vi "Measurement UI.vi"() -> ()   [LabVIEW 2023, in "Single Tone_Class D Amplifier_UI.lvlib"]
uses:
  Single Tone_Class D Amplifier_UI.lvlib
  shared/controls/units - snr.ctl
  shared/controls/units - ratio.ctl
  shared/controls/digital output level units.ctl
  shared/ui/controls/view.ctl
  UI State.ctl
  <vilib>/Utility/miscctls.llb/LVBoundsTypeDef.ctl
  <vilib>/Utility/miscctls.llb/LVPoint32TypeDef.ctl
  <vilib>/Utility/miscctls.llb/LVPointTypeDef.ctl
  shared/ui/UI Helpers.lvlib
  shared/audio popup ui/Audio Popup UI.lvlib
  shared/controls/audio controls.lvlib
panel:
  in  "view legend":T1
  out "time domain":waveform(dbl)[](graph)
  out "frequency domain":cluster{"x0":dbl, "dx":dbl, "magnitude":dbl[]}[](graph)
  out "meas table":string[][](table)
  in  "digital serial cfg file":string
  out "output power (W)":dbl[](array[numeric])
  out "SFDR (dBc)":dbl[](array[numeric])
  out "gain":dbl[](array[numeric])
  out "dynamic range (dB)":dbl[](array[numeric])
  out "THD":dbl[](array[numeric])
  out "THD+N":dbl[](array[numeric])
  out "SNR":dbl[](array[numeric])
  out "phase (deg)":dbl[](array[numeric])
  out "amplitude (dBFS)":dbl[](array[numeric])
  out "amplitude (Vrms)":dbl[](array[numeric])
  out "frequency (Hz)":dbl[](array[numeric])
  out "channel names":string[](array[string])
  in  "Configuration tab":enum32{"Protocol", "Measurement", "Units"}(tab)
  out "digital serial file name":string
  in  "configure digital serial":bool
  in  "master clock channel list":string caption="Master Clock Channel"
  in  "digital channel list":string caption="Digital Audio Channel"
  in  "output level":dbl=-1.0 caption="Output level" format="%#_3f"
  in  "output level units":T2
  in  "min settling cycles":u32 caption="Minimum settling cycles"
  in  "min settling time (s)":dbl=0.1 caption="Minimum settling time" format="%#_6ps"
  in  "min measurement cycles":u32 caption="Minimum measurement cycles"
  in  "min measurement time (s)":dbl=0.1 caption="Minimum measurement time" format="%#_6ps"
  in  "Acquisition channel":tag
  in  "acq sampling rate":dbl=51200.0 caption="Sample rate" format="%#.6pHz"
  in  "lowpass filter":T3(ring) caption="Lowpass filter"
  in  "highpass filter":enum32{"DC", "AC"}(ring) caption="Highpass filter"
  in  "band start":dbl=20.0 caption="Band start" format="%#_6pHz"
  in  "band stop":dbl=20000.0 caption="Band stop" format="%#_6pHz"
  in  "weighting filter":T4(ring)=enum."A-weighting" caption="Weighting filter"
  in  "load impedance":dbl=4.0 caption="Load impedance" format="%#_6p Ohms"
  in  "output range (pk-pk)":dbl=15.0 caption="Output range" format="%.3p Vpk-pk"
  in  "signal frequency":dbl=1000.0 caption="Frequency" format="%#_6pHz"
  in  "gain units":T5 caption="Gain"
  in  "THD units":T5 caption="THD"
  in  "THD+N units":T5 caption="THD+N"
  in  "SNR units":T6 caption="SNR"
  in  "channel 0 offset":u32=1
  out "fft - data":dbl[](array[numeric])
  out "fft - df":dbl
  out "fft - f0":dbl
  out "wfm - data":dbl[](array[numeric])
  out "wfm - dt":dbl
  out "wfm - t0":dbl
  in  "acq channel":string="PXI1Slot4/ai0"
  in  "signal phase":dbl caption="phase"
  # "hidden controls - used to sync with MeasLink"
  # "hidden indicators"
  # "Digital Serial Settings"
  # "Harware Resource"
  # "Filters"
  # "Output"
  # "Acquisition"
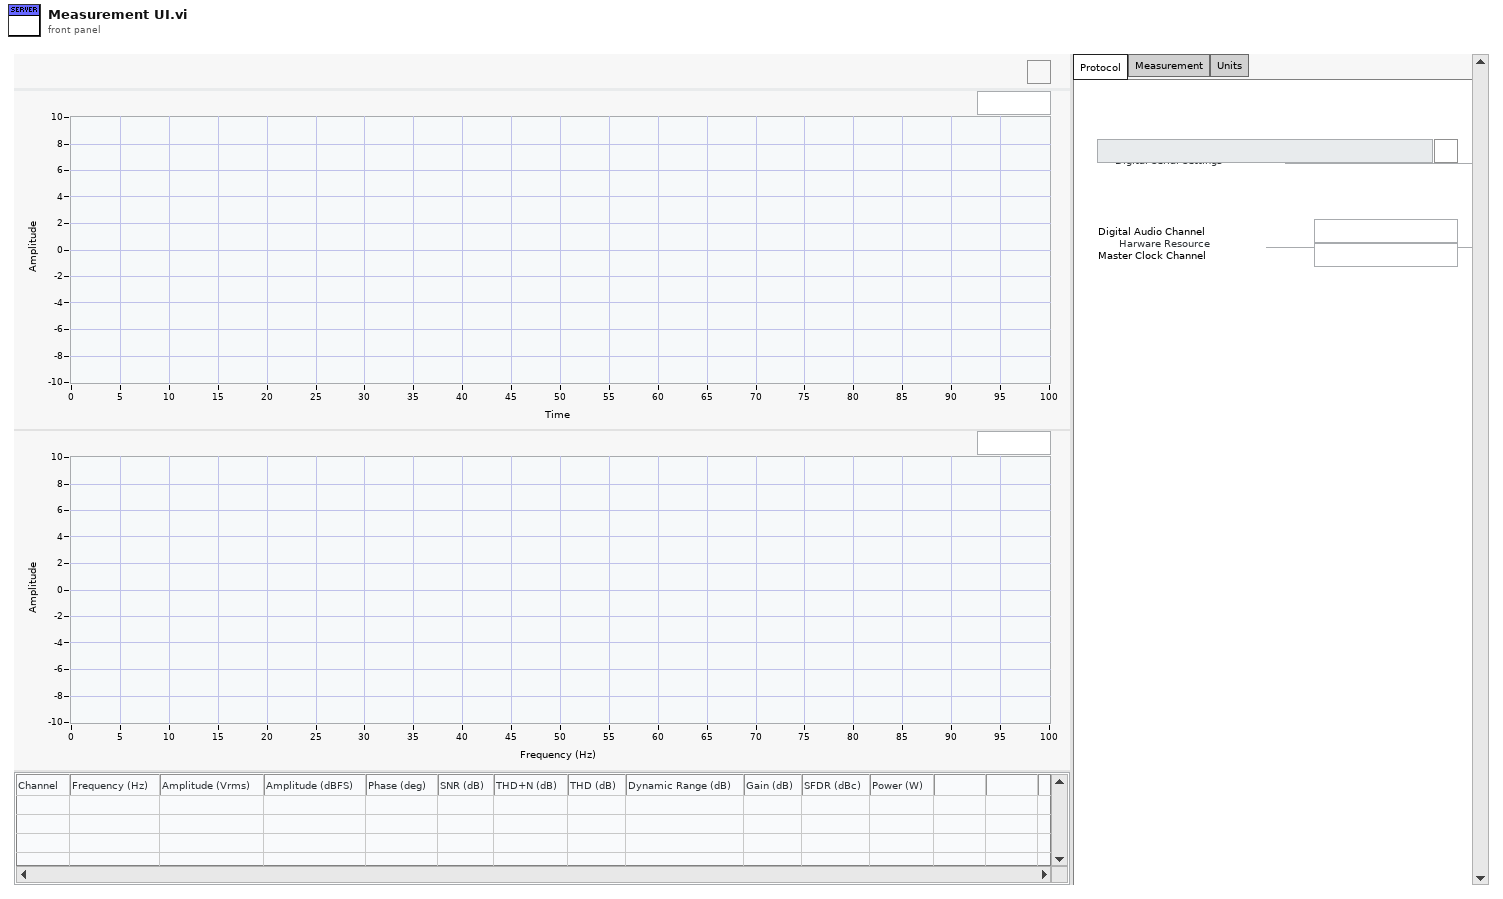
[diagram p1: front panel]
types:
  T1 = typedef "UI Helpers.lvlib/view.ctl" = bool
  T2 = typedef "audio controls.lvlib/digital output level units.ctl" = enum32{"% FS", "dBFS", "V"}
  T3 = enum32{"No filter", "AES17 20kHz", "AES17 40kHz"}
  T4 = enum32{"Linear", "A-weighting", "B-weighting", "C-weighting"}
  T5 = typedef "audio controls.lvlib/units - ratio.ctl" = enum32{"dB", "%", "x/y"}
  T6 = typedef "audio controls.lvlib/units - snr.ctl" = enum32{"dB", "x/y"}
  T7 = typedef "Single Tone_Class D Amplifier_UI.lvlib/UI State.ctl" = cluster{"Graph Size":T8, "Legend Visible":bool, "Mouse Coords":T9, "PostUI event occurred":bool, "digital serial cfg file":path}
  T8 = typedef "LVBoundsTypeDef.ctl" = cluster{"Width":u32, "Height":u32}
  T9 = typedef "LVPoint32TypeDef.ctl" = cluster{"Horizontal":i32, "Vertical":i32}
  T10 = typedef "LVPointTypeDef.ctl" = cluster{"Horizontal":i16, "Vertical":i16}
  T11 = typedef "Audio Popup UI.lvlib/audio settings.ctl" = cluster{"digital serial file":string}
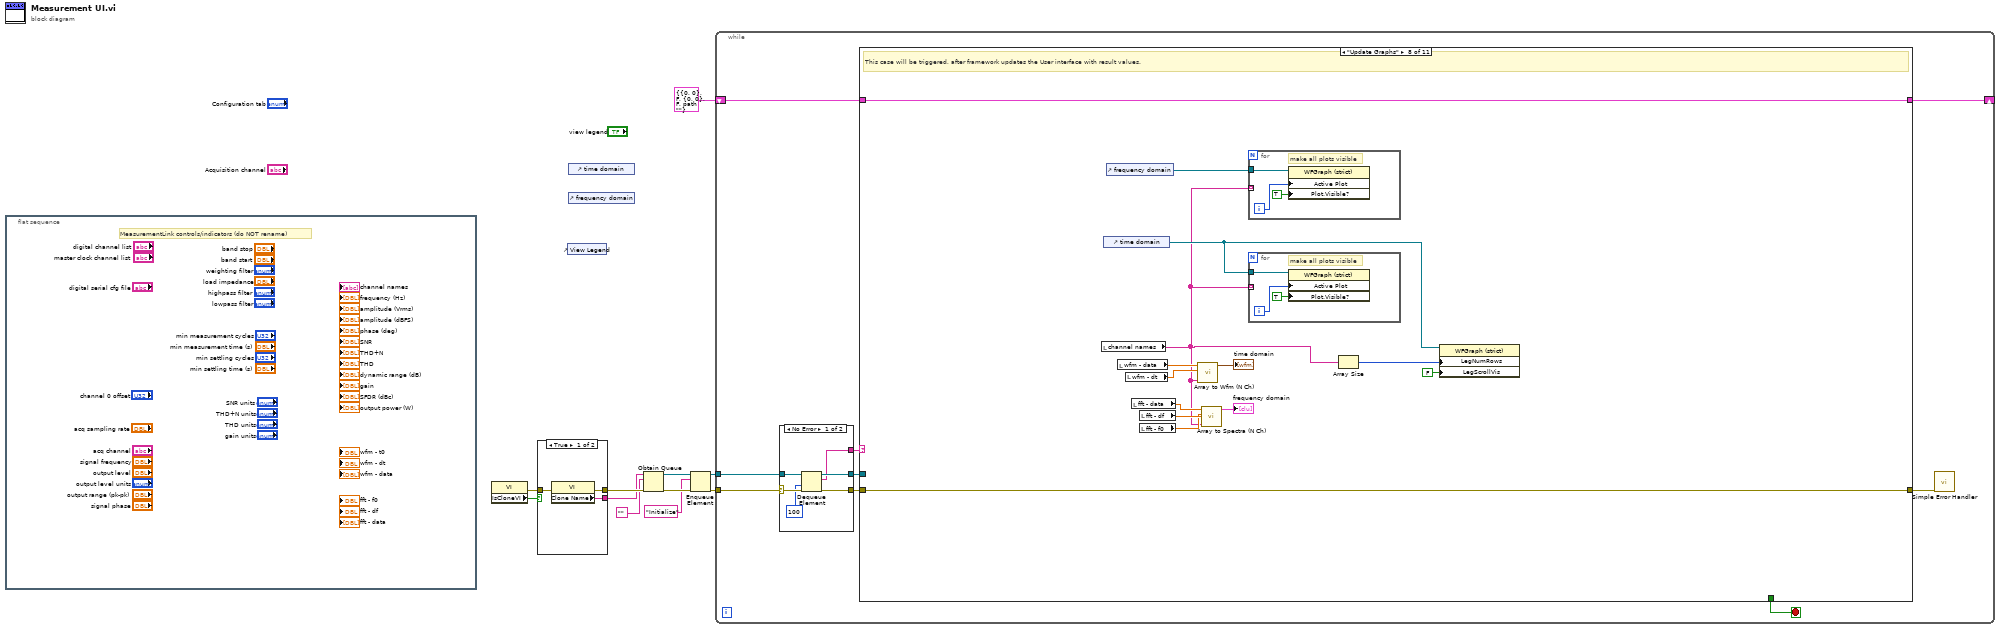
[diagram p0: block diagram]
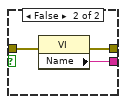
[diagram p2: hidden frame]
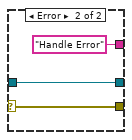
[diagram p3: hidden frame]
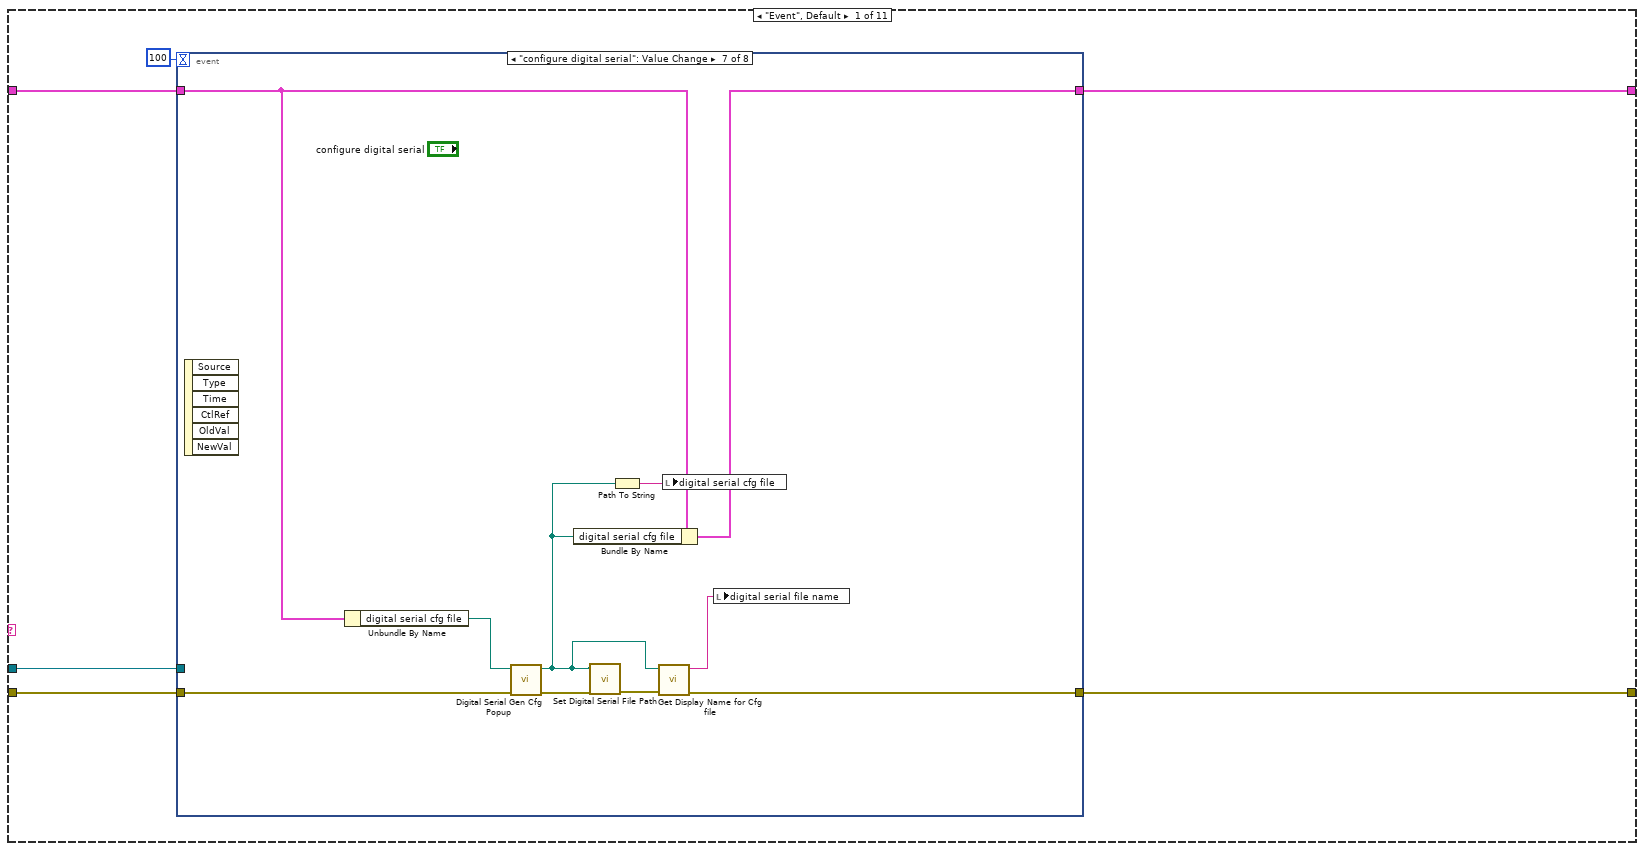
[diagram p4: hidden frame]
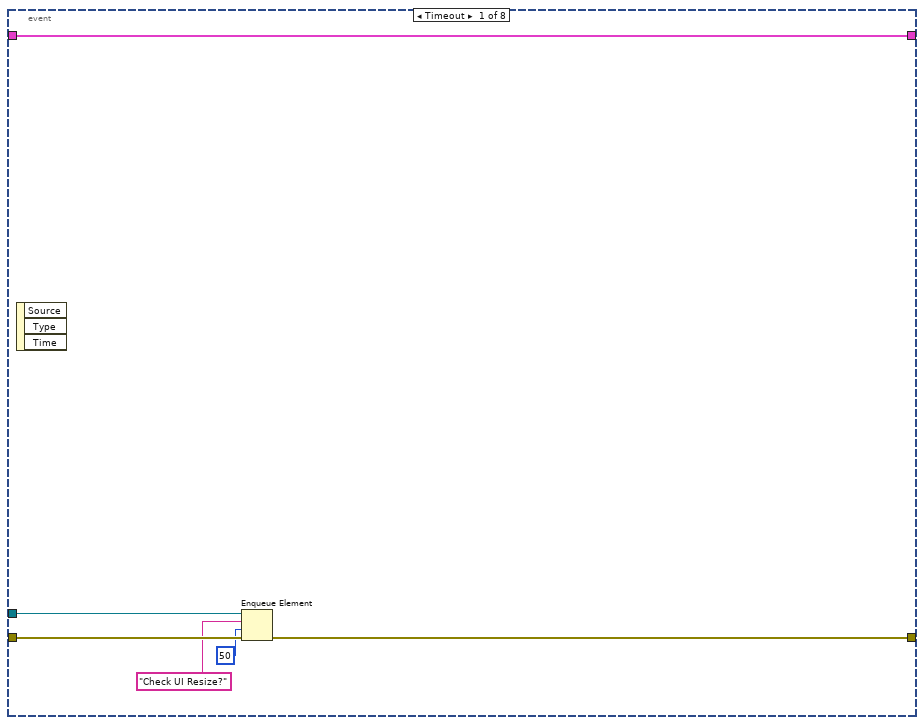
[diagram p5: hidden frame]
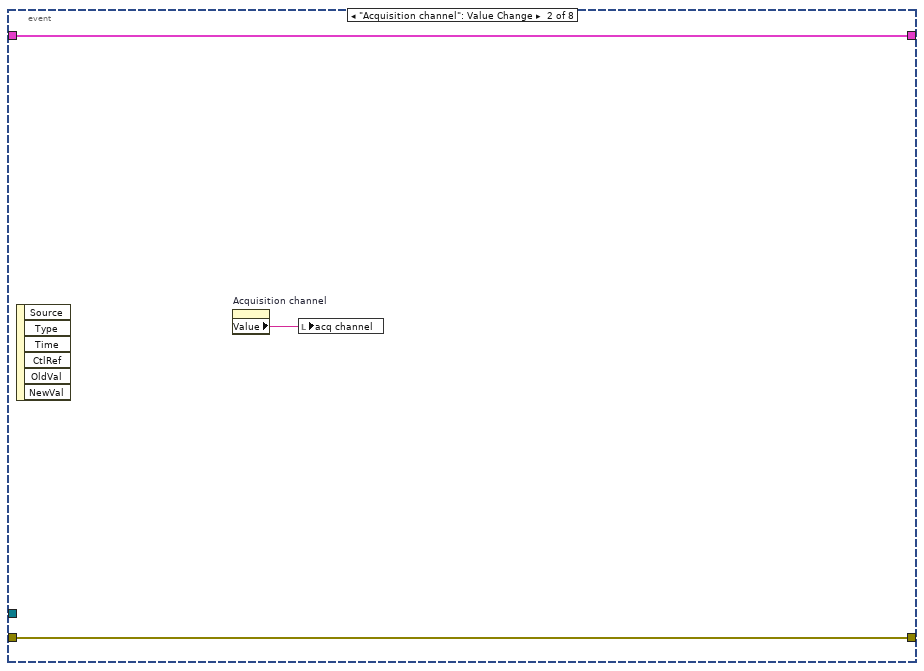
[diagram p6: hidden frame]
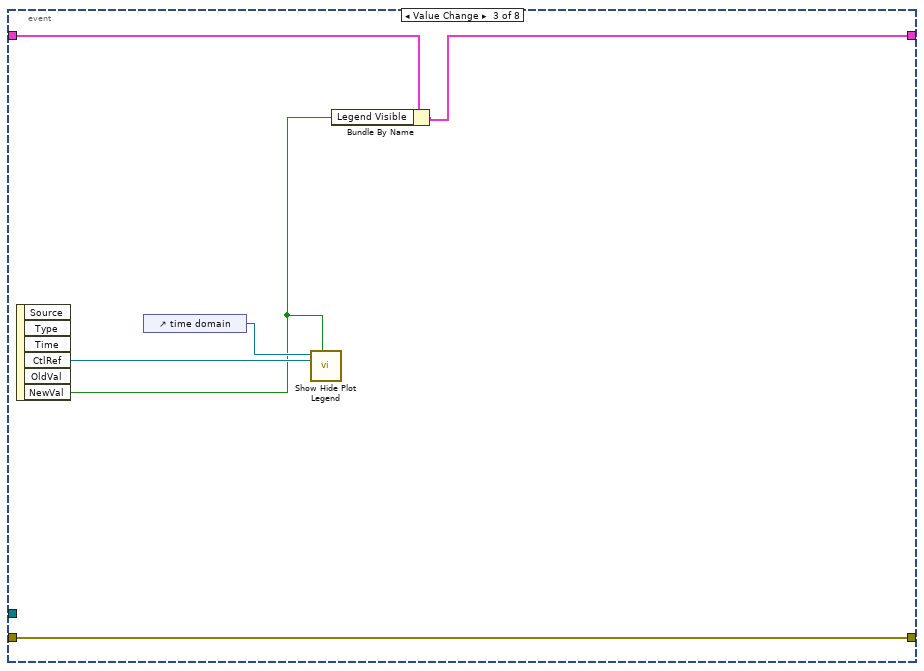
[diagram p7: hidden frame]
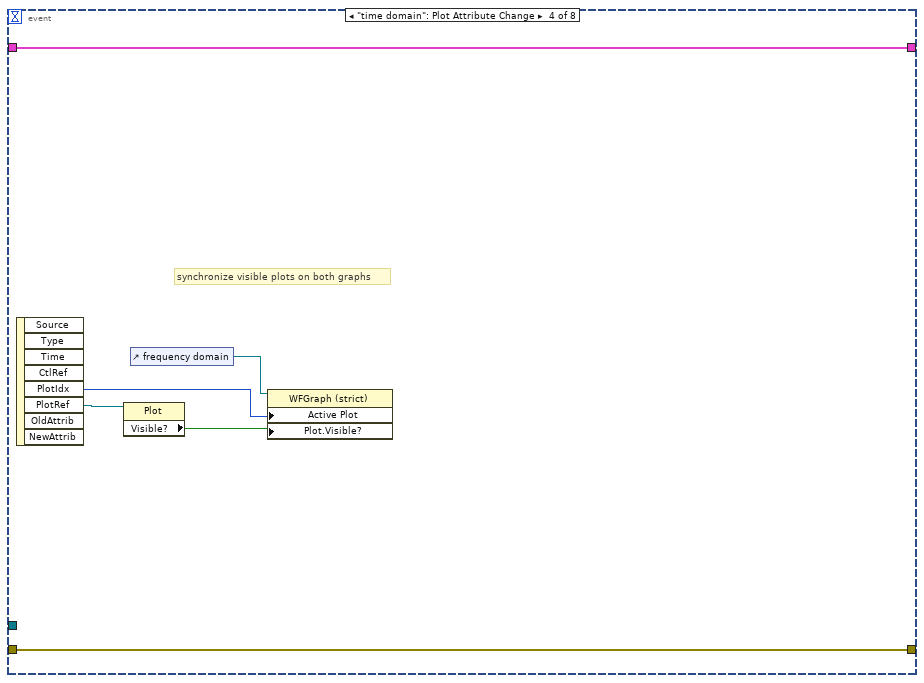
[diagram p8: hidden frame]
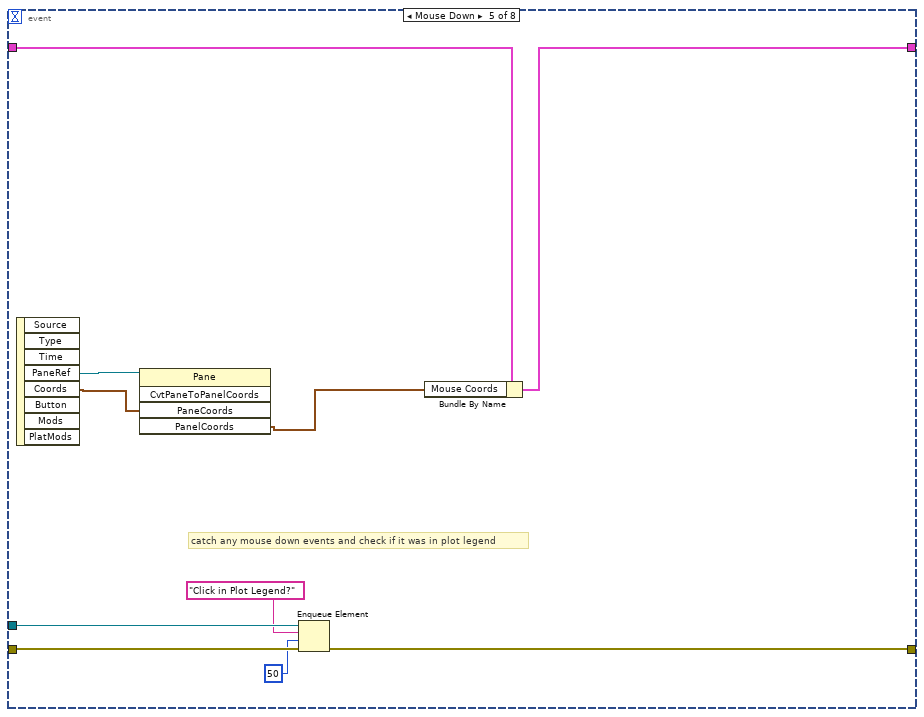
[diagram p9: hidden frame]
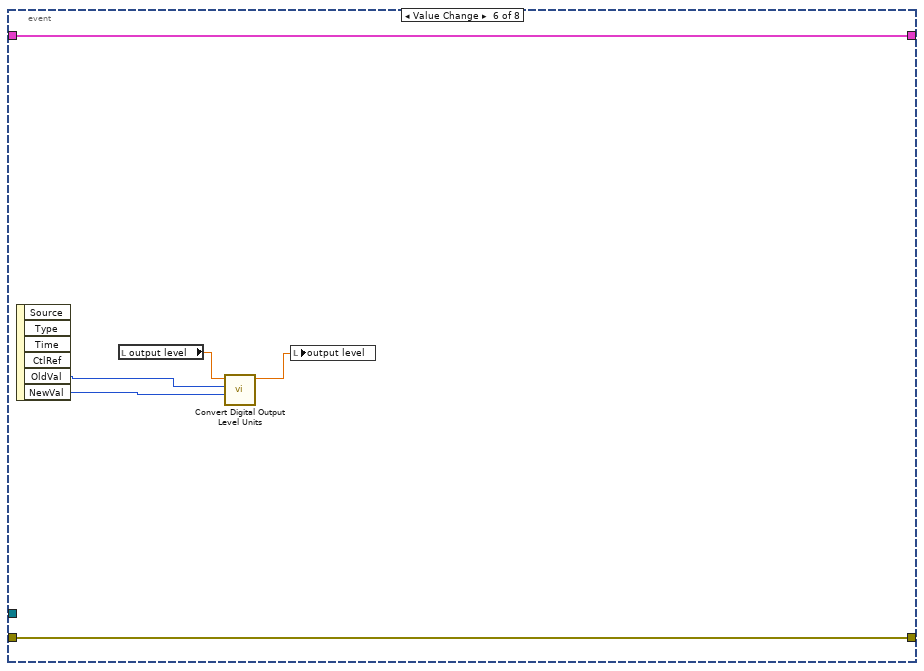
[diagram p10: hidden frame]
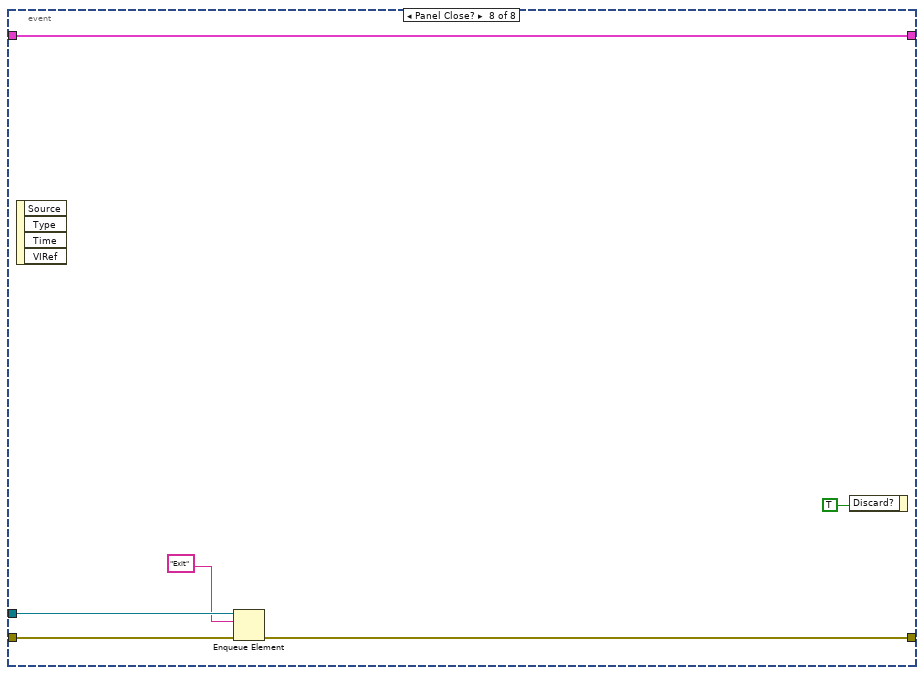
[diagram p11: hidden frame]
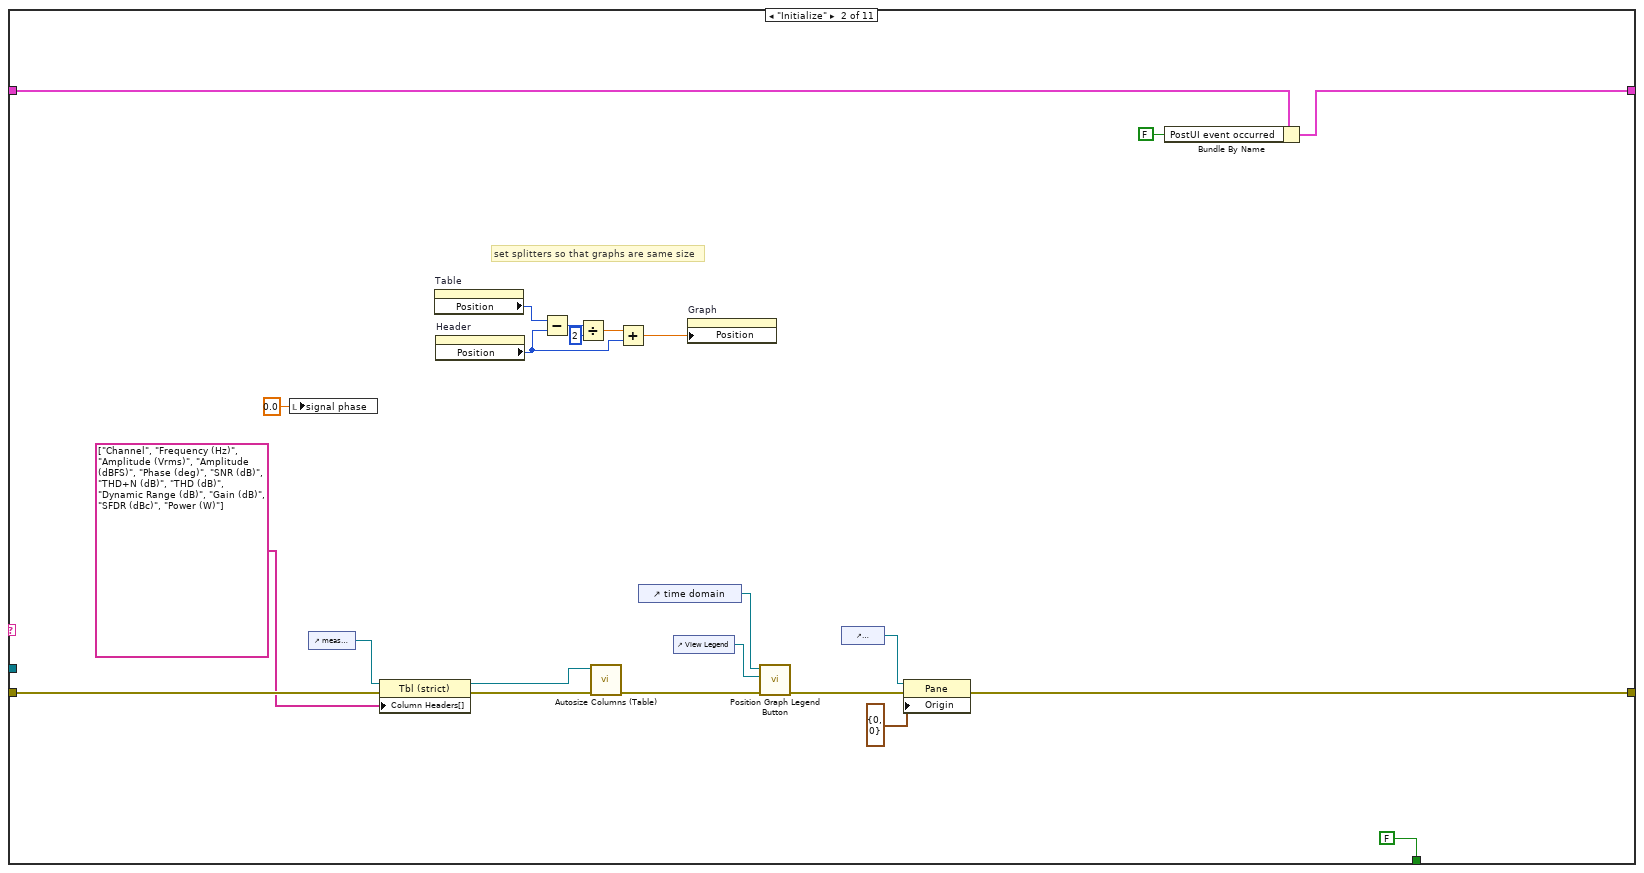
[diagram p12: hidden frame]
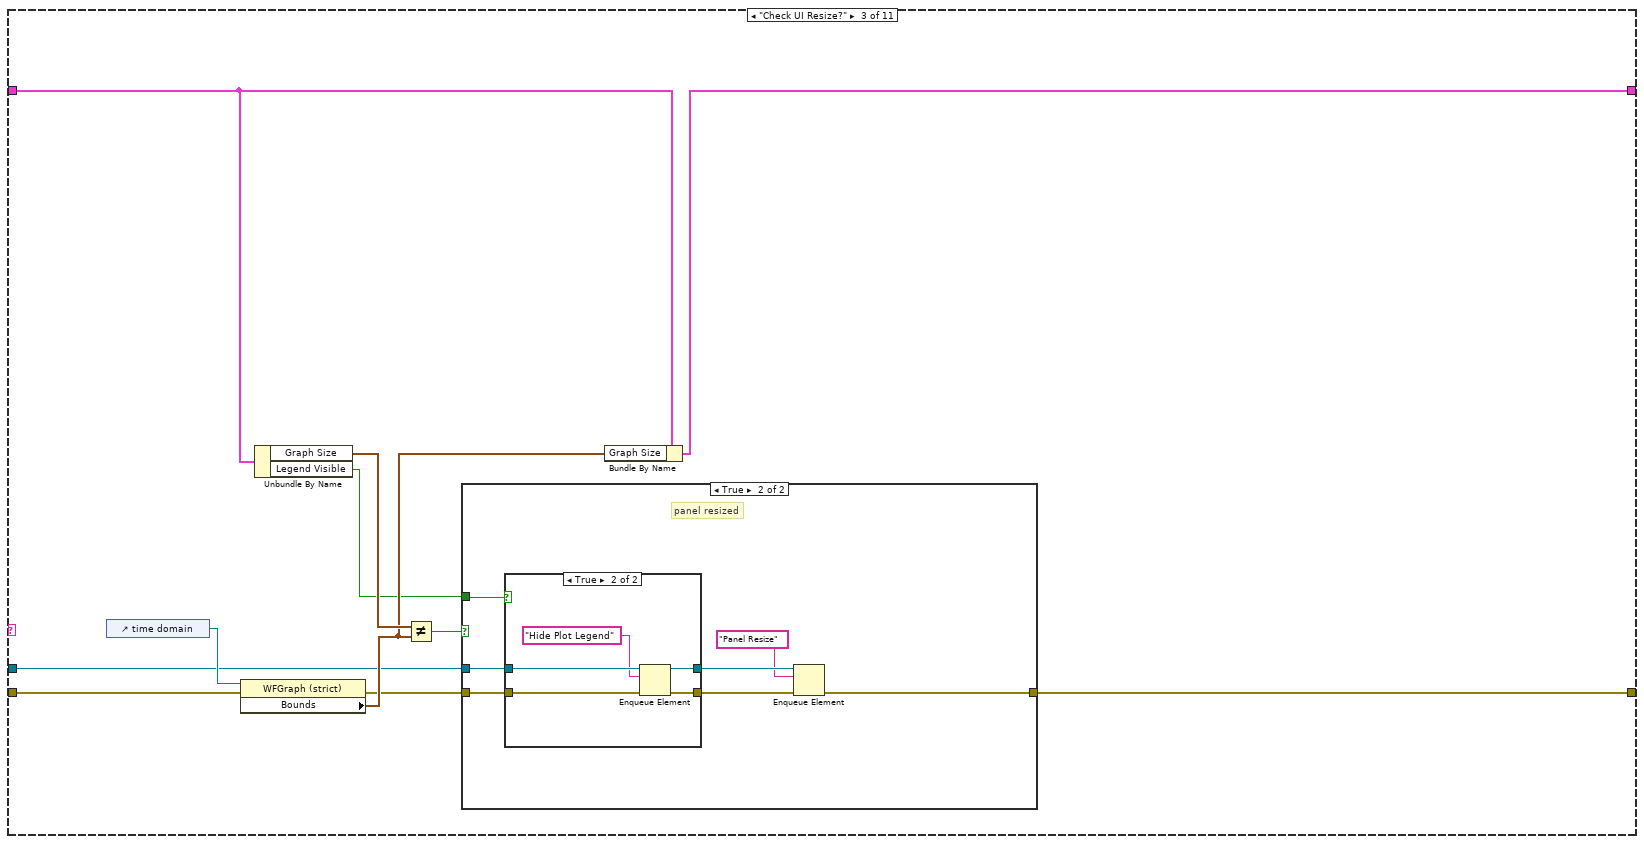
[diagram p13: hidden frame]
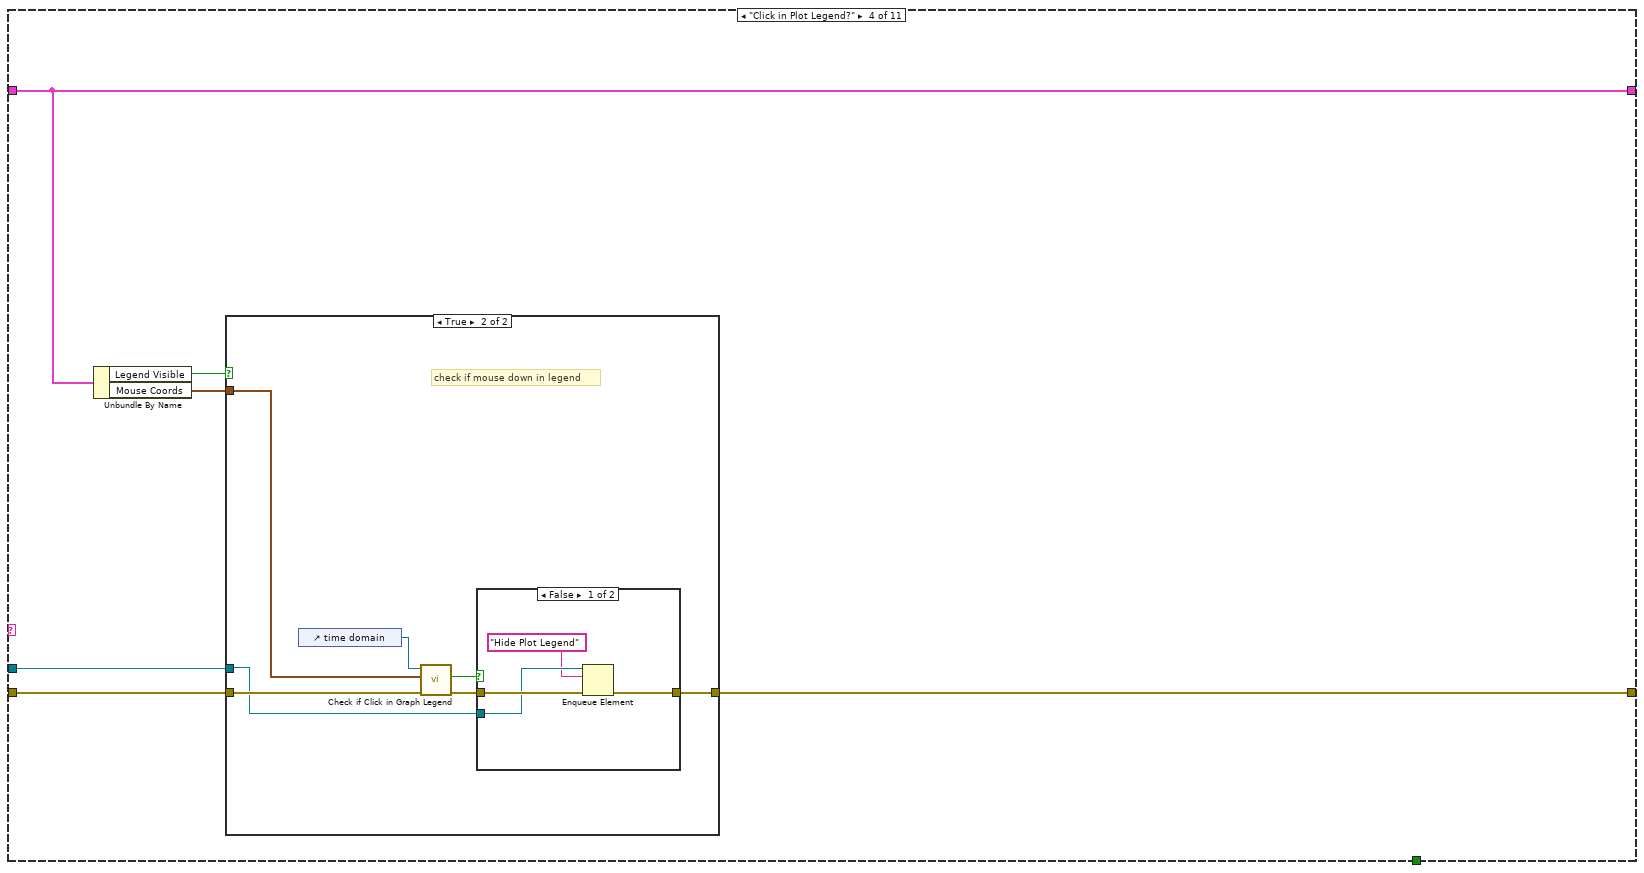
[diagram p16: hidden frame]
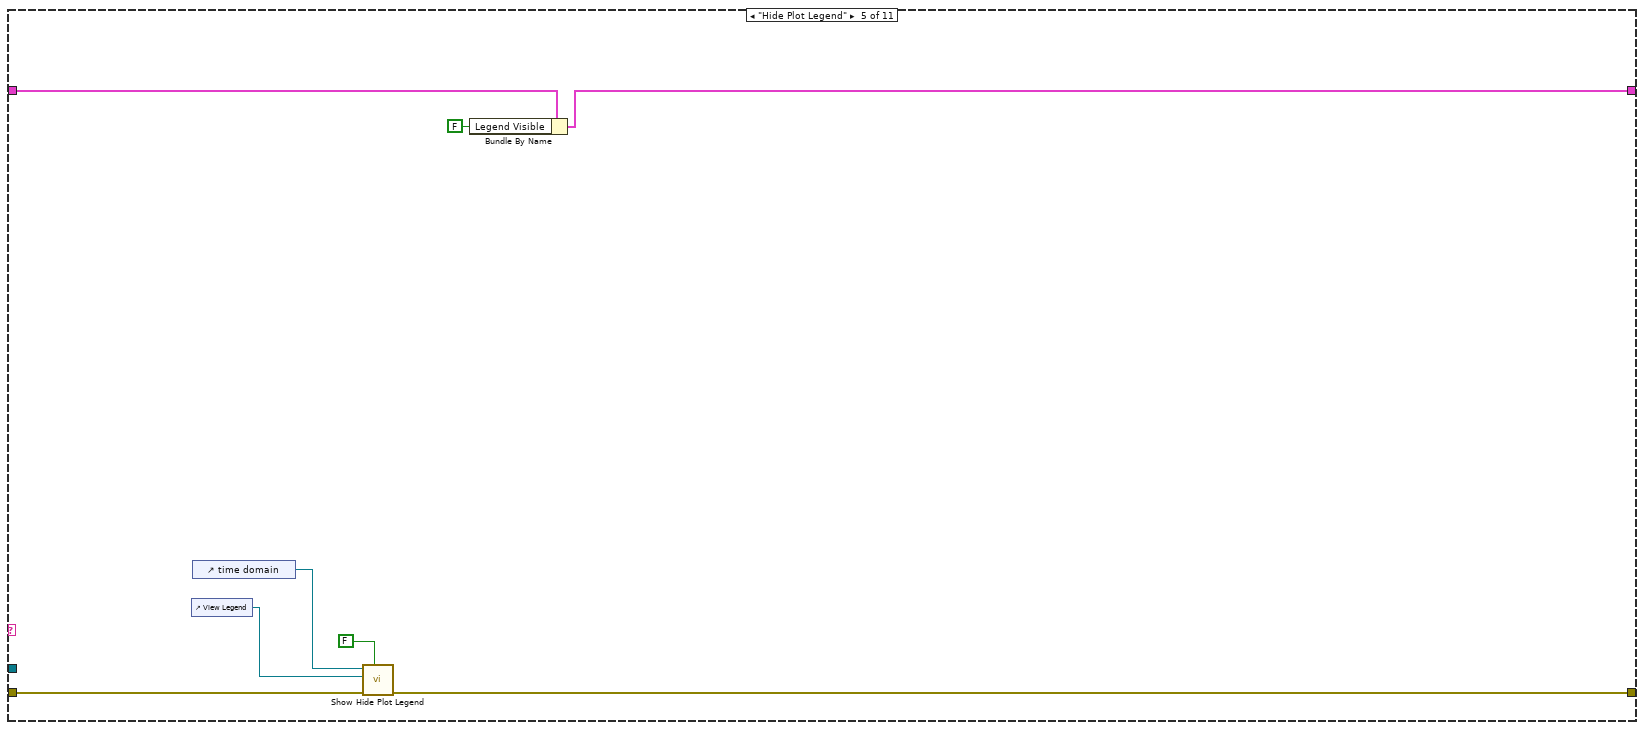
[diagram p19: hidden frame]
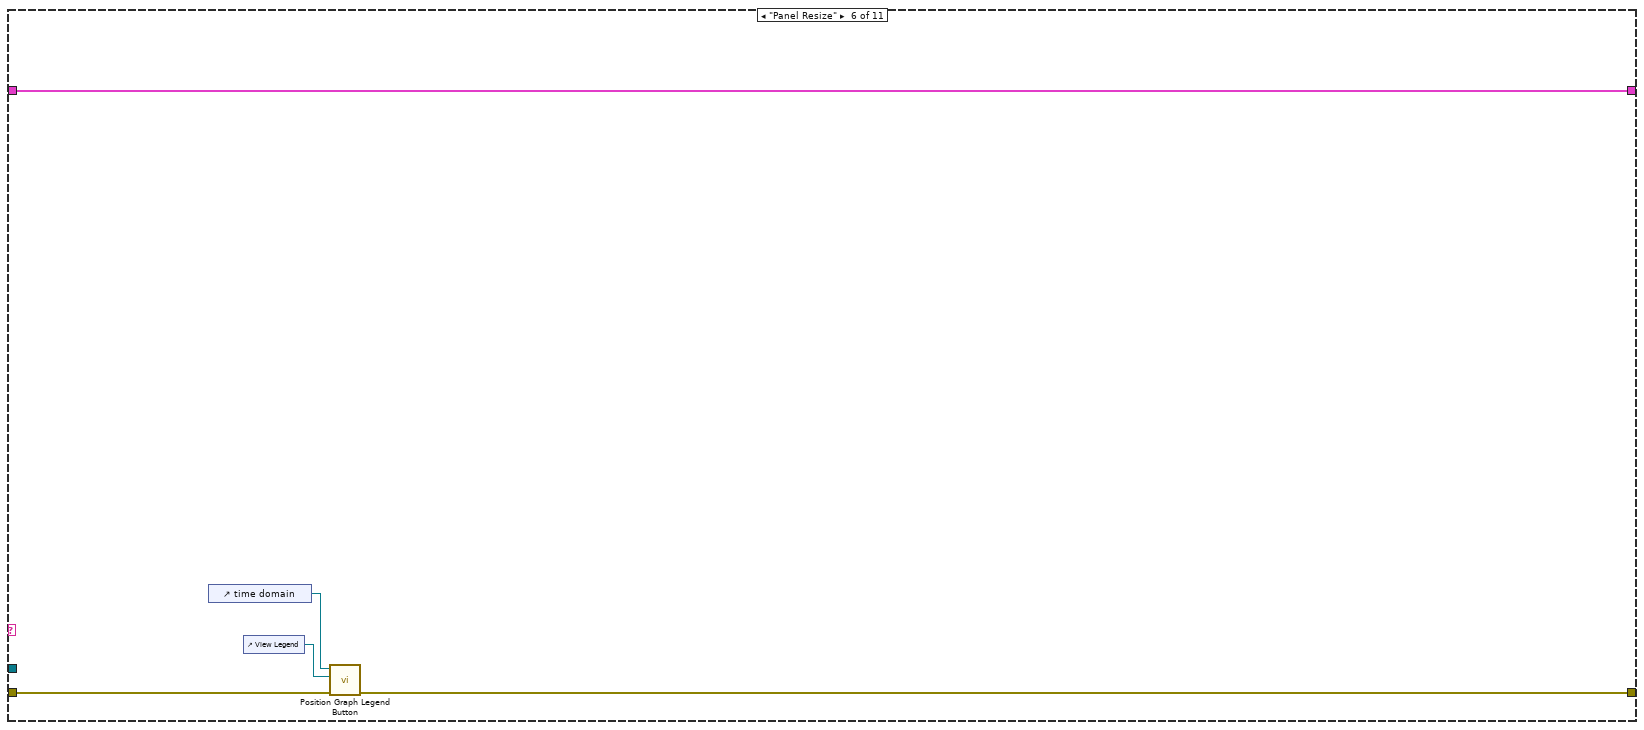
[diagram p20: hidden frame]
diagram:
  n1 = flat-sequence {
    frame #0 {
      # "MeasurementLink controls/indicators (do NOT rename)"
    }
  }
  n2 = property class="VI"() -> (error out=w2:errorcluster, "IsCloneVI"=w3:bool)  [unwired: 2 in, 1 out]
  n3 = case shown="True" w3 {
    tunnel: [w14 w17] -> w11
    tunnel: [w13 w16] -> w10
    tunnel: w2 -> [w12 w15]
    frame True {
      n4 = property class="VI"(error in=w12) -> (error out=w14:errorcluster, "Clone Name"=w13:string)  [unwired: 1 in, 1 out]
    }
    frame False {
      n5 = property class="VI"(error in=w15) -> (error out=w17:errorcluster, "Name"=w16:string)  [unwired: 1 in, 1 out]
    }
  }
  n6 = control-ref of="View Legend"() -> ()  [unwired: 1 out]
  n7 = control-ref of="time domain"() -> ()  [unwired: 1 out]
  n8 = control-ref of="frequency domain"() -> ()  [unwired: 1 out]
  n9 = Obtain Queue(name (unnamed)=w10, element data type="", error in (no error)=w11) -> (queue out=w7:refnum<queue>, error out=w9:errorcluster)  [unwired: 2 in, 1 out]
  n10 = Enqueue Element(queue=w7, element="Initialize", error in (no error)=w9) -> (queue out=w6:refnum<queue>, error out=w8:errorcluster)  [unwired: 1 in, 1 out]
  n11 = while {
    tunnel: w6 -> [w24]
    shift-right: [w20] -> _
    shift-left: T7 {"Graph Size"={"Width"=0, "Height"=0}, "Legend Visible"=FALSE, "Mouse Coords"={"Horizontal"=0, "Vertical"=0}, "PostUI event occurred"=FALSE, "digital serial cfg file"=path ""} ("ui state") -> [w19]
    tunnel: w8 -> [w26]
    stop <- w21 stop-if-true
    n12 = case shown="No Error" w26 {
      selector: w26 -> [w32 w35]
      tunnel: [w31 w35] -> w25
      tunnel: w24 -> [w30 w34]
      tunnel: [w29 w34] -> w23
      tunnel: [w28 "Handle Error"] -> w22
      frame No Error {
        n13 = Dequeue Element(queue=w30, timeout in ms (-1)=100, error in (no error)=w32) -> (queue out=w29:refnum<queue>, element=w28:string, error out=w31:errorcluster)  [unwired: 1 out]
      }
      frame Error {
      }
    }
    n14 = case shown="\"Update Graphs\"" w22 {
      tunnel: w25 -> [w40 w112 w127 w145 w167 w172 w183 w221 w229 w355 w357]
      tunnel: w23 -> [w38 _ w118 w146 _ _ w182 _ _ w353 _]
      tunnel: [w41 w98 w120 w144 w166 w171 w178 w221 w233 w350 w357] -> w18
      tunnel: [_ FALSE _ _ _ _ _ _ _ TRUE _] -> w21
      tunnel: [w36 w96 w123 w149 w168 w175 w176 w222 w230 w348 w356] -> w20
      tunnel: w19 -> [w37 w97 w124 w149 w169 w175 w177 w222 w230 w348 w356]
      frame "Event", Default {
        n15 = event shown="[6] \"configure digital serial\": Value Change" {
          selector: _ -> [_ _ _ _ _ _ _ _]
          dyn-events: _ -> [_ _ _ _ _ _ _ _]
          timeout: 100 -> [_ _ _ _ _ _ _ _]
          tunnel: [w44 w48 w53 w57 w70 w73 w79 w92] -> w41
          tunnel: w40 -> [w47 w48 w53 w57 w71 w73 w88 w93]
          tunnel: w38 -> [w46 _ _ _ w72 _ _ w91]
          tunnel: w37 -> [w43 w49 w55 w58 w67 w74 w85 w89]
          tunnel: [w43 w49 w54 w58 w66 w74 w84 w89] -> w36
          event Timeout {
            n16 = event-data() -> ()  [unwired: 1 in, 3 out]
            n17 = Enqueue Element(queue=w46, element="Check UI Resize?", timeout in ms (-1)=50, error in (no error)=w47) -> (error out=w44:errorcluster)  [unwired: 2 out]
          }
          event "Acquisition channel": Value Change {
            n18 = event-data() -> ()  [unwired: 1 in, 6 out]
            n19 = property on="Acquisition channel" class="DAQmxName"() -> ("Value"=w50:string)  [unwired: 2 in, 2 out]
            n20 = local write "acq channel"(w50) -> ()
          }
          event Value Change {
            n21 = event-data() -> ("CtlRef"=w52:refnum<vi>, "NewVal"=w51:T1)  [unwired: 1 in, 4 out]
            n22 = control-ref of="time domain"() -> (w56:refnum<vi>)
            n23 = call "Show Hide Plot Legend.vi"("show"=w51, "view reference"=w52, "graph reference"=w56) -> ()  [unwired: 8 in, 1 out]
            n24 = Bundle By Name(cluster=w55, "Legend Visible"=w51) -> (w54:T7)
          }
          event "time domain": Plot Attribute Change {
            # "synchronize visible plots on both graphs"
            n25 = event-data() -> ("PlotIdx"=w60:i32, "PlotRef"=w61:refnum<vi>)  [unwired: 1 in, 6 out]
            n26 = property class="Plot"(reference=w61) -> ("Visible?"=w62:bool)  [unwired: 1 in, 2 out]
            n27 = control-ref of="frequency domain"() -> (w59:refnum<vi>)
            n28 = property on="Property Node" class="WFGraph (strict)"(reference=w59, "Active Plot"=w60, "Plot.Visible?"=w62) -> ()  [unwired: 1 in, 2 out]
          }
          event Mouse Down {
            # "catch any mouse down events and check if it was in plot legend"
            n29 = event-data() -> ("PaneRef"=w65:refnum<vi>, "Coords"=w64:T9)  [unwired: 1 in, 6 out]
            n30 = invoke class="Pane" method="CvtPaneToPanelCoords"(reference=w65, "PaneCoords"=w64) -> ("PanelCoords"=w63:T10)  [unwired: 3 in, 4 out]
            n31 = Enqueue Element(queue=w72, element="Click in Plot Legend?", timeout in ms (-1)=50, error in (no error)=w71) -> (error out=w70:errorcluster)  [unwired: 2 out]
            n32 = Bundle By Name(cluster=w67, "Mouse Coords"=w63) -> (w66:T7)
          }
          event Value Change {
            n33 = event-data() -> ("OldVal"=w78:T2, "NewVal"=w77:T2)  [unwired: 1 in, 4 out]
            n34 = local read "output level"() -> (w76:dbl)
            n35 = call "Convert Digital Output Level Units.vi"("new output level units"=w77, "previous output level units"=w78, "previous output level"=w76) -> ("new output level"=w75:dbl)  [unwired: 8 in]
            n36 = local write "output level"(w75) -> ()
          }
          event "configure digital serial": Value Change {
            n37 = event-data() -> ()  [unwired: 1 in, 6 out]
            n38 = Unbundle By Name(w85) -> ("digital serial cfg file"=w86:path)
            n39 = call "Digital Serial Gen Cfg Popup.vi"("error in (no error)"=w88, "config file in"=w86) -> ("error out"=w82:errorcluster, "config file out"=w81:path)  [unwired: 7 in, 1 out]
            n40 = Bundle By Name(cluster=w85, "digital serial cfg file"=w81) -> (w84:T7)
            n41 = call "Set Digital Serial File Path.vi"("error in (no error)"=w82, "digital serial file"=w81) -> ("error out"=w80:errorcluster)  [unwired: 9 in]
            n42 = Path To String(path=w81) -> (string=w87:string)
            n43 = call "Get Display Name for Cfg file.vi"("error in (no error)"=w80, "file path"=w81) -> ("error out"=w79:errorcluster, "display string"=w83:string)  [unwired: 8 in]
            n44 = local write "digital serial cfg file"(w87) -> ()
            n45 = local write "digital serial file name"(w83) -> ()
          }
          event Panel Close? {
            n46 = event-data() -> ()  [unwired: 1 in, 4 out]
            n47 = Enqueue Element(queue=w91, element="Exit", error in (no error)=w93) -> (error out=w92:errorcluster)  [unwired: 1 in, 2 out]
            n48 = event-data("Discard?"=TRUE) -> ()  [unwired: 1 in, 1 out]
          }
        }
      }
      frame "Initialize" {
        # "set splitters so that graphs are same size"
        n49 = local write "signal phase"(0.0 ("signal phase")) -> ()
        n50 = control-ref of="meas table"() -> (w110:refnum<vi>)
        n51 = property class="Tbl (strict)"(reference=w110, error in=w112, "Column Headers[]"=string[] ["Channel", "Frequency (Hz)", "Amplitude (Vrms)", "Amplitude (dBFS)", "Phase (deg)", "SNR (dB)", "THD+N (dB)", "THD (dB)", "Dynamic Range (dB)", "Gain (dB)", "SFDR (dBc)", "Power (W)"] ("Column Header Strings[]")) -> (reference out=w109:refnum<vi>, error out=w111:errorcluster)
        n52 = property on="Table" class="Splitter"() -> ("Position"=w107:i32)  [unwired: 2 in, 2 out]
        n53 = property on="Header" class="Splitter"() -> ("Position"=w103:i32)  [unwired: 2 in, 2 out]
        n54 = Subtract(x=w107, y=w103) -> (x-y=w106:i32)
        n55 = Divide(x=w106, y=2) -> (x/y=w104:dbl)
        n56 = call "Autosize Columns (Table).vi"("error in (no error)"=w111, "table"=w109) -> ("error out"=w113:errorcluster)  [unwired: 9 in]
        n57 = Add(x=w104, y=w103) -> (x+y=w102:dbl)
        n58 = control-ref of="time domain"() -> (w115:refnum<vi>)
        n59 = control-ref of="View Legend"() -> (w114:refnum<vi>)
        n60 = property on="Graph" class="Splitter"("Position"=w102) -> ()  [unwired: 2 in, 2 out]
        n61 = call "Position Graph Legend Button.vi"("error in (no error)"=w113, "view legend"=w114, "graph"=w115) -> ("error out"=w101:errorcluster)  [unwired: 8 in]
        n62 = control-ref of="Configuration"() -> (w100:refnum<vi>)
        n63 = property class="Pane"(reference=w100, error in=w101, "Origin"=T10 {"Horizontal"=0, "Vertical"=0}) -> (error out=w98:errorcluster)  [unwired: 1 out]
        n64 = Bundle By Name(cluster=w97, "PostUI event occurred"=FALSE) -> (w96:T7)
      }
      frame "Check UI Resize?" {
        n65 = control-ref of="time domain"() -> (w128:refnum<vi>)
        n66 = property on="Property Node" class="WFGraph (strict)"(reference=w128, error in=w127) -> (error out=w121:errorcluster, "Bounds"=w125:T8)  [unwired: 1 out]
        n67 = Unbundle By Name(w124) -> ("Graph Size"=w126:T8, "Legend Visible"=w119:bool)
        n68 = Not Equal?(x=w126, y=w125) -> (x != y?=w122:bool)
        n69 = case shown="True" w122 {
          tunnel: w121 -> [w129 w136]
          tunnel: [w129 w131] -> w120
          tunnel: w119 -> [_ w134]
          tunnel: w118 -> [_ w135]
          frame False {
            # "no resize"
          }
          frame True {
            # "panel resized"
            n70 = case shown="True" w134 {
              tunnel: w136 -> [w138 w143]
              tunnel: [w138 w142] -> w133
              tunnel: w135 -> [w137 w141]
              tunnel: [w137 w139] -> w132
              frame False {
              }
              frame True {
                n71 = Enqueue Element(queue=w141, element="Hide Plot Legend", error in (no error)=w143) -> (queue out=w139:refnum<queue>, error out=w142:errorcluster)  [unwired: 1 in, 1 out]
              }
            }
            n72 = Enqueue Element(queue=w132, element="Panel Resize", error in (no error)=w133) -> (error out=w131:errorcluster)  [unwired: 1 in, 2 out]
          }
        }
        n73 = Bundle By Name(cluster=w124, "Graph Size"=w125) -> (w123:T7)
      }
      frame "Click in Plot Legend?" {
        n74 = Unbundle By Name(w149) -> ("Legend Visible"=w148:bool, "Mouse Coords"=w147:T9)
        n75 = case shown="True" w148 {
          tunnel: w147 -> [_ w155]
          tunnel: w146 -> [_ w152]
          tunnel: w145 -> [w150 w157]
          tunnel: [w150 w151] -> w144
          frame False {
            # "legend not visible; do nothing"
          }
          frame True {
            # "check if mouse down in legend"
            n76 = control-ref of="time domain"() -> (w156:refnum<vi>)
            n77 = call "Check if Click in Graph Legend.vi"("error in (no error)"=w157, "Mouse Coords"=w155, "WaveformGraph"=w156) -> ("error out"=w153:errorcluster, "click in legend?"=w154:bool)  [unwired: 7 in]
            n78 = case shown="False" w154 {
              tunnel: w153 -> [w161 w162]
              tunnel: w152 -> [w160 _]
              tunnel: [w159 w162] -> w151
              frame False {
                n79 = Enqueue Element(queue=w160, element="Hide Plot Legend", error in (no error)=w161) -> (error out=w159:errorcluster)  [unwired: 1 in, 2 out]
              }
              frame True {
                # "inside legend; do nothing"
              }
            }
          }
        }
      }
      frame "Hide Plot Legend" {
        n80 = control-ref of="View Legend"() -> (w163:refnum<vi>)
        n81 = control-ref of="time domain"() -> (w164:refnum<vi>)
        n82 = call "Show Hide Plot Legend.vi"("show"=FALSE, "error in (no error)"=w167, "view reference"=w163, "graph reference"=w164) -> ("error out"=w166:errorcluster)  [unwired: 7 in]
        n83 = Bundle By Name(cluster=w169, "Legend Visible"=FALSE ("legend visible")) -> (w168:T7)
      }
      frame "Panel Resize" {
        n84 = control-ref of="time domain"() -> (w174:refnum<vi>)
        n85 = control-ref of="View Legend"() -> (w173:refnum<vi>)
        n86 = call "Position Graph Legend Button.vi"("error in (no error)"=w172, "view legend"=w173, "graph"=w174) -> ("error out"=w171:errorcluster)  [unwired: 8 in]
      }
      frame "Post UI Update" {
        # "This case will be triggered, after framework updates the User interface with result values."
        n87 = for {
          tunnel: w182 -> [w206]
          shift-right: [w205] -> w179
          shift-left: w183 -> [w207]
          tunnel: string[] ["Update Table", "Update Graphs"] -> [w204] mode=indexing
          n88 = Enqueue Element(queue=w206, element=w204, timeout in ms (-1)=50, error in (no error)=w207) -> (error out=w205:errorcluster)  [unwired: 2 out]
        }
        n89 = Unbundle By Name(w177) -> ("PostUI event occurred"=w180:bool)
        n90 = case shown="False" w180 {
          tunnel: w179 -> [w190 w203]
          tunnel: [w185 w203] -> w178
          tunnel: w177 -> [w193 w202]
          tunnel: [w192 w202] -> w176
          frame False {
            # "do this on first PostUI Event (happens when panel loads)"
            # "Initialize the DAQmx channel control"
            n91 = local read "digital serial cfg file"() -> (w189:string)
            n92 = local read "acq channel"() -> (w195:string)
            n93 = property on="Acquisition channel" class="DAQmxName"("Value"=w195) -> ()  [unwired: 2 in, 2 out]
            n94 = Empty String/Path?(string/path=w189) -> (empty?=w191:bool)
            n95 = case shown="True" w191 {
              tunnel: w190 -> [w197 w201]
              tunnel: [w197 w199] -> w188
              tunnel: w189 -> [w196 _]
              tunnel: [w196 w198] -> w184
              frame False {
              }
              frame True {
                n96 = call "Get Audio Settings.vi"("error in (no error)"=w201) -> ("error out"=w199:errorcluster, "audio settings"=w200:T11)  [unwired: 9 in]
                n97 = Unbundle By Name(w200) -> ("digital serial file"=w198:string)
              }
            }
            n98 = String To Path(string=w184) -> (path=w187:path)
            n99 = call "Get Display Name for Cfg file.vi"("error in (no error)"=w188, "file path"=w187) -> ("error out"=w185:errorcluster, "display string"=→"digital serial file name":string)  [unwired: 8 in]
            n100 = local write "digital serial cfg file"(w184) -> ()
            n101 = Bundle By Name(cluster=w193, "PostUI event occurred"=TRUE, "digital serial cfg file"=w187) -> (w192:T7)
          }
          frame True {
          }
        }
      }
      frame "Update Graphs" {
        # "This case will be triggered, after framework updates the User interface with result values."
        n102 = local read "channel names"() -> (w210:string[])
        n103 = control-ref of="time domain"() -> (w213:refnum<vi>)
        n104 = control-ref of="frequency domain"() -> (w209:refnum<vi>)
        n105 = local read "wfm - data"() -> (w220:dbl[])
        n106 = local read "wfm - dt"() -> (w219:dbl)
        n107 = local read "fft - data"() -> (w217:dbl[])
        n108 = local read "fft - df"() -> (w216:dbl)
        n109 = local read "fft - f0"() -> (w215:dbl)
        n110 = call "Array to Wfm (N Ch).vi"("channel names"=w210, "dt"=w219, "array"=w220) -> ("waveforms"=→"time domain":waveform(dbl)[])  [unwired: 8 in]
        n111 = call "Array to Spectra (N Ch).vi"("channel names"=w210, "df"=w216, "f0"=w215, "data"=w217) -> ("spectra"=→"frequency domain":cluster{"f0":dbl, "df":dbl, "data":dbl[]}[])  [unwired: 7 in]
        n112 = for {
          tunnel: w209 -> [w223]
          tunnel: w210 -> [_] mode=indexing
          i -> [w224]
          # "make all plots visible"
          n113 = property class="WFGraph (strict)"(reference=w223, "Active Plot"=w224, "Plot.Visible?"=TRUE ("Plot.Visible")) -> ()  [unwired: 1 in, 2 out]
        }
        n114 = for {
          tunnel: w213 -> [w226]
          tunnel: w210 -> [_] mode=indexing
          i -> [w227]
          # "make all plots visible"
          n115 = property class="WFGraph (strict)"(reference=w226, "Active Plot"=w227, "Plot.Visible?"=TRUE ("Plot.Visible")) -> ()  [unwired: 1 in, 2 out]
        }
        n116 = Array Size(array=w210) -> (size(s)=w212:i32)
        n117 = property class="WFGraph (strict)"(reference=w213, "LegNumRows"=w212, "LegScrollVis"=FALSE ("Legend:Scrollbar Visible")) -> ()  [unwired: 1 in, 2 out]
      }
      frame "Update Table" {
        # "format data for table"
        # "This case will be triggered, after framework updates the User interface with result values."
        n118 = local read "SNR units"() -> (w273:T6)
        n119 = local read "gain units"() -> (w269:T5)
        n120 = local read "THD+N units"() -> (w285:T5)
        n121 = local read "THD units"() -> (w271:T5)
        n122 = case shown="\"x/y\"" w273 {
          tunnel: ["(dB)" "(ratio)"] -> w284
          tunnel: ["%5.1f" ("initial string") "%.1f" ("initial string")] -> w267
          frame "dB", Default {
          }
          frame "x/y" {
          }
        }
        n123 = case shown="\"x/y\"" w285 {
          tunnel: ["(dB)" "(%)" "(ratio)"] -> w287
          tunnel: ["%5.1f" ("initial string") "%.3f" ("initial string") "%.6f" ("initial string")] -> w264
          frame "dB", Default {
          }
          frame "%" {
          }
          frame "x/y" {
          }
        }
        n124 = case shown="\"x/y\"" w271 {
          tunnel: ["(dB)" "(%)" "(ratio)"] -> w272
          tunnel: ["%5.1f" ("initial string") "%.3f" ("initial string") "%.6f" ("initial string")] -> w261
          frame "dB", Default {
          }
          frame "%" {
          }
          frame "x/y" {
          }
        }
        n125 = case shown="\"%\"" w269 {
          tunnel: ["(dB)" "(%)" "(ratio)"] -> w270
          tunnel: ["%5.1f" ("initial string") "%.1f" ("initial string") "%.3f" ("initial string")] -> w251
          frame "dB", Default {
          }
          frame "%" {
          }
          frame "x/y" {
          }
        }
        n126 = Concatenate Strings("SNR " ("string"), w284) -> (w281:string)
        n127 = Concatenate Strings("THD+N " ("string"), w287) -> (w280:string)
        n128 = Concatenate Strings("Gain " ("string"), w270) -> (w278:string)
        n129 = Concatenate Strings("THD " ("string"), w272) -> (w279:string)
        n130 = property on="meas table" class="Tbl (strict)"() -> ("Column Headers[]"=w234:string[])  [unwired: 2 in, 2 out]
        n131 = Replace Array Subset(array=w234, new element #1=w281, index #1=5 ("index"), new element #2=w280, index #2=6 ("index"), new element #3=w279, index #3=7 ("index"), new element #4=w278, index #4=9 ("index")) -> (w282:string[])
        n132 = property on="meas table" class="Tbl (strict)"("Column Headers[]"=w282) -> ()  [unwired: 2 in, 2 out]
        n133 = local read "amplitude (Vrms)"() -> (w246:dbl[])
        n134 = local read "amplitude (dBFS)"() -> (w243:dbl[])
        n135 = local read "frequency (Hz)"() -> (w249:dbl[])
        n136 = local read "phase (deg)"() -> (w239:dbl[])
        n137 = local read "THD+N"() -> (w266:dbl[])
        n138 = local read "THD"() -> (w263:dbl[])
        n139 = local read "SNR"() -> (w268:dbl[])
        n140 = local read "channel names"() -> (w231:string[])
        n141 = for {
          tunnel: [w304] -> w248 mode=indexing
          tunnel: w249 -> [w303] mode=indexing
          tunnel: "%.3f" ("initial string") -> [w302]
          n142 = Format Into String(format string=w302, w303) -> (resulting string=w304:string)  [unwired: 2 in, 1 out]
        }
        n143 = for {
          tunnel: [w301] -> w245 mode=indexing
          tunnel: w246 -> [w300] mode=indexing
          tunnel: "%.3f" ("initial string") -> [w299]
          n144 = Format Into String(format string=w299, w300) -> (resulting string=w301:string)  [unwired: 2 in, 1 out]
        }
        n145 = for {
          tunnel: [w298] -> w242 mode=indexing
          tunnel: w243 -> [w297] mode=indexing
          tunnel: "%.3f" ("initial string") -> [w296]
          n146 = Format Into String(format string=w296, w297) -> (resulting string=w298:string)  [unwired: 2 in, 1 out]
        }
        n147 = for {
          tunnel: [w319] -> w262 mode=indexing
          tunnel: w263 -> [w318] mode=indexing
          tunnel: w261 -> [w317]
          n148 = Format Into String(format string=w317, w318) -> (resulting string=w319:string)  [unwired: 2 in, 1 out]
        }
        n149 = for {
          tunnel: [w325] -> w257 mode=indexing
          tunnel: w268 -> [w324] mode=indexing
          tunnel: w267 -> [w323]
          n150 = Format Into String(format string=w323, w324) -> (resulting string=w325:string)  [unwired: 2 in, 1 out]
        }
        n151 = for {
          tunnel: [w322] -> w265 mode=indexing
          tunnel: w266 -> [w321] mode=indexing
          tunnel: w264 -> [w320]
          n152 = Format Into String(format string=w320, w321) -> (resulting string=w322:string)  [unwired: 2 in, 1 out]
        }
        n153 = for {
          tunnel: [w295] -> w240 mode=indexing
          tunnel: w239 -> [w294] mode=indexing
          tunnel: "%.3f" ("initial string") -> [w293]
          n154 = Format Into String(format string=w293, w294) -> (resulting string=w295:string)  [unwired: 2 in, 1 out]
        }
        n155 = local read "dynamic range (dB)"() -> (w259:dbl[])
        n156 = local read "output power (W)"() -> (w255:dbl[])
        n157 = local read "SFDR (dBc)"() -> (w253:dbl[])
        n158 = local read "gain"() -> (w252:dbl[])
        n159 = for {
          tunnel: [w316] -> w258 mode=indexing
          tunnel: w259 -> [w315] mode=indexing
          tunnel: "%5.1f" ("initial string") -> [w314]
          n160 = Format Into String(format string=w314, w315) -> (resulting string=w316:string)  [unwired: 2 in, 1 out]
        }
        n161 = for {
          tunnel: [w307] -> w238 mode=indexing
          tunnel: w252 -> [w306] mode=indexing
          tunnel: w251 -> [w305]
          n162 = Format Into String(format string=w305, w306) -> (resulting string=w307:string)  [unwired: 2 in, 1 out]
        }
        n163 = for {
          tunnel: [w310] -> w237 mode=indexing
          tunnel: w253 -> [w309] mode=indexing
          tunnel: "%5.1f" ("initial string") -> [w308]
          n164 = Format Into String(format string=w308, w309) -> (resulting string=w310:string)  [unwired: 2 in, 1 out]
        }
        n165 = for {
          tunnel: [w313] -> w236 mode=indexing
          tunnel: w255 -> [w312] mode=indexing
          tunnel: "%.3f" ("initial string") -> [w311]
          n166 = Format Into String(format string=w311, w312) -> (resulting string=w313:string)  [unwired: 2 in, 1 out]
        }
        n167 = Build Array(w231, w248, w245, w242, w240, w257, w265, w262, w258, w238, w237, w236) -> (w235:string[][])
        n168 = Transpose 2D Array(2D array=w235) -> (transposed array=w232:string[][])
        "meas table" <- w232
        n169 = flat-sequence {
          tunnel: [w292] -> w233
          tunnel: w232 -> [_]
          tunnel: w229 -> [w290]
          frame #0 {
            n170 = control-ref of="meas table"() -> (w291:refnum<vi>)
            n171 = call "Autosize Columns (Table).vi"("error in (no error)"=w290, "table"=w291) -> ("error out"=w292:errorcluster)  [unwired: 9 in]
          }
        }
      }
      frame "Exit" {
        # "This case is triggered to close the User Interface from framework"
        n172 = Flush Queue(queue=w353, error in (no error)=w355) -> (queue out=w352:refnum<queue>, error out=w351:errorcluster)  [unwired: 1 out]
        n173 = Release Queue(queue=w352, force destroy? (F)=TRUE, error in (no error)=w351) -> (error out=w350:errorcluster)  [unwired: 2 out]
      }
      frame "Handle Error" {
      }
    }
    n174 = call <vilib>:"Simple Error Handler.vi"("error in (no error)"=w18) -> ()  [unwired: 4 in, 5 out]
  }
